vi "Logging_PathConfig.vi"() -> (5 "Front panel image path":path, 6 "Log File path":path, 7 "Model path":path)   [LabVIEW 2020]
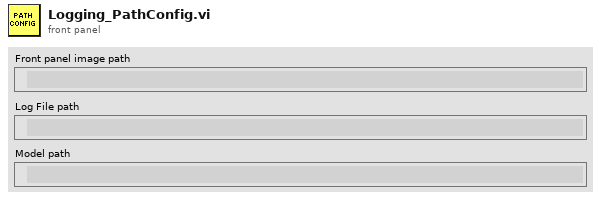
[diagram p1: front panel]
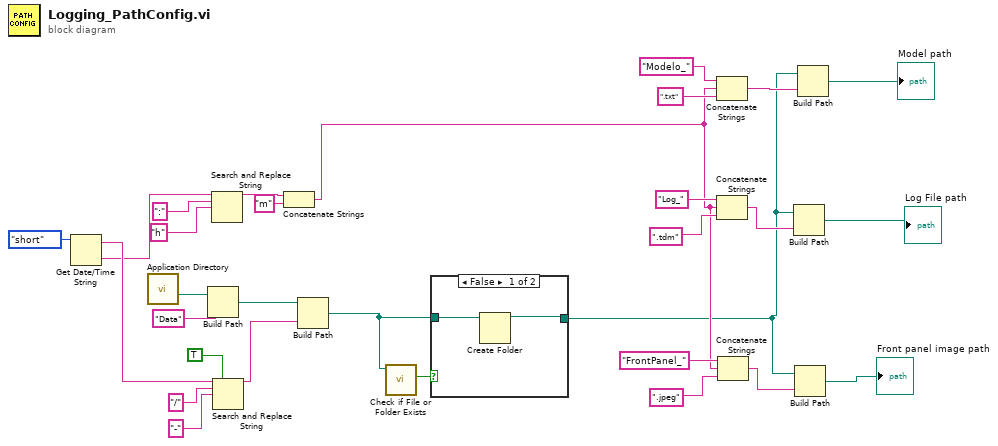
[diagram p0: block diagram]
diagram:
  n1 = Get Date/Time String(date format (0)=enum16{"short", "long", "abbreviated"}."short") -> (date string=w18:string, time string=w5:string)  [unwired: 2 in]
  n2 = call <vilib>:"Application Directory.vi"() -> ("Application Directory"=w22:path)
  n3 = Build Path(base path=w22, name or relative path="Data") -> (appended path=w20:path)
  n4 = Search and Replace String(input string=w5, search string=":", replace string="h" ("replace string (\"\")")) -> (result string=w7:string)  [unwired: 5 in, 3 out]
  n5 = Search and Replace String(replace all?=TRUE ("replace all? (F)"), input string=w18, search string="/", replace string="-" ("replace string (\"\")")) -> (result string=w14:string)  [unwired: 4 in, 3 out]
  n6 = Concatenate Strings(w7, "m" ("string")) -> (w4:string)
  n7 = Build Path(base path=w20, name or relative path=w14) -> (appended path=w2:path)
  n8 = call <vilib>:"Check if File or Folder Exists.vi"("path"=w2) -> ("file or folder exists?"=w3:bool)  [unwired: 8 in, 2 out]
  n9 = case shown="False" w3 {
    tunnel: [w31 w33] -> w1
    tunnel: w2 -> [w32 w33]
    frame False {
      n10 = Create Folder(path (use dialog)=w32) -> (created path=w31:path)  [unwired: 2 in, 2 out]
    }
    frame True {
    }
  }
  n11 = Concatenate Strings("Modelo_" ("string"), w4, ".txt" ("string")) -> (w29:string)
  n12 = Concatenate Strings("Log_" ("string"), w4, ".tdm" ("string")) -> (w24:string)
  n13 = Concatenate Strings("FrontPanel_" ("string"), w4, ".jpeg" ("string")) -> (w12:string)
  n14 = Build Path(base path=w1, name or relative path=w24) -> (appended path=→"Log File path":path)
  n15 = Build Path(base path=w1, name or relative path=w12) -> (appended path=→"Front panel image path":path)
  n16 = Build Path(base path=w1, name or relative path=w29) -> (appended path=→"Model path":path)
